vi "DeppGetRegRepeat.vi"(7 "Overlap?":bool, 8 "Error In":errorcluster, 9 "Num Bytes":u32, 10 "Address":u8, 11 "Device Handle":u32) -> (0 "Error Out":errorcluster, 2 "Data":u8[](array[numeric]), 3 "Device Handle":u32)   [LabVIEW 2011, in "LVH-Adept.lvlib" / "DEPP.lvlib"]
uses:
  <vilib>/LabVIEW Hacker/Adept/Private/DEPP/DEPP.lvlib
  <vilib>/LabVIEW Hacker/Adept/Private/DEPP/Private/Type Defs/Error.ctl
  <vilib>/LabVIEW Hacker/Adept/Private/Resources/depp.dll
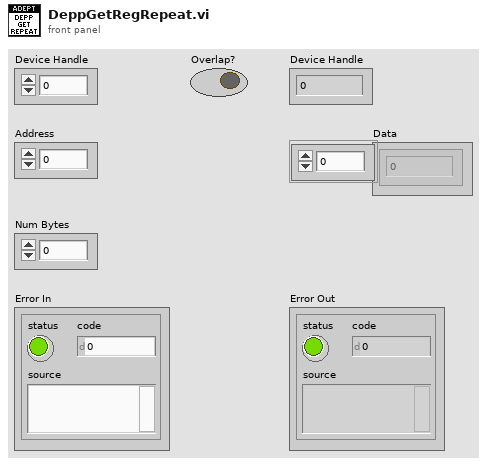
[diagram p1: front panel]
types:
  T1 = typedef "LVH-Adept.lvlib/DEPP.lvlib/Error.ctl" = enum16{"Unknown", "Enable", "Get Register", "Get Register Repeat", "Get Register Set", "Put Register", "Put Register Repeat", "Put Register Set", "Disable", "Set Pair Size"}
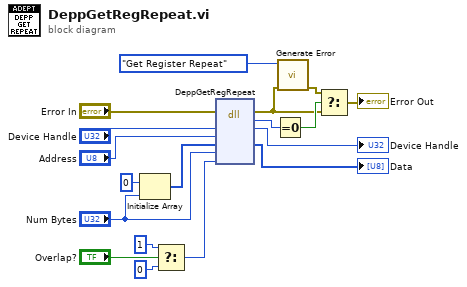
[diagram p0: block diagram]
diagram:
  n1 = Initialize Array(u8 0 ("t"), "Num Bytes") -> (w3:u8[])
  n2 = Select(t=u8 1, s="Overlap?", f=u8 0) -> (s? t:f=w5:u8)
  n3 = dll-call lib="C:/Program Files (x86)/National Instruments/LabVIEW 2011/vi.lib/LabVIEW Hacker/Adept/Private/Resources/depp.dll" fn="DeppGetRegRepeat"(error in="Error In", "hif"="Device Handle", "bAddr"="Address", "pbData"=w3, "cbData"="Num Bytes", "fOverlap"=w5) -> (error out=w10:errorcluster, "Success"=w17:u32, "hif"=→"Device Handle":u32, "pbData"=→"Data":u8[])  [unwired: 5 in, 1 out]
  n4 = Equal To 0?(x=w17) -> (x = 0?=w16:bool)
  n5 = call <vilib>:"Generate Error.vi"("Error In"=w10, "DEPP Error"=Error."Get Register Repeat") -> ("Error Out"=w11:errorcluster)  [unwired: 9 in]
  n6 = Select(t=w11, s=w16, f=w10) -> (s? t:f=→"Error Out":errorcluster)
